vi "HapticSPM_write_test-bench.vi"() -> ()   [LabVIEW 2022 SP3]
uses:
  <vilib>/Utility/sysdir.llb/System Directory Type.ctl
  Haptic-Programming-Interface/LabVIEW VIs/Haptic Prog Interface/Haptic Prog Interface.lvlib
panel:
  out "Signal & Force (Scaled)":dbl[][](graph)
  out "Force vs Signal":cluster{dbl[], dbl[]}(graph)
  in  "Stop":bool
  in  "Mode Selection":string(combo)="2" caption="Combo Box"
  in  "Suggested Settings":bool=TRUE
  in  "Cursor":bool=TRUE
  out "?":bool=TRUE
  out "data":dbl[][](array[numeric])
  in  "Tab Control":enum32{"2 atoms", "1 atom", "Line", "N"}(tab)
  out "Frame Properties (m)":T1
  in  "Function":string(combo)="0" caption="Combo Box"
  in  "Gain (mm/pm)":dbl=2.0 caption="Numeric" format="%.1g"
  in  "k":dbl=0.6000000000000001 caption="Numeric" step=0.1 format="%.1g"
  in  "Setpoint":dbl=8.000000413701856e-11 caption="Numeric" step=1e-11 format="%.0p"
  in  "Gain":dbl=1.0 caption="Numeric" format="%.1g"
  out "Value":dbl caption="Numeric" format="%#_2p"
  out "Click Number":dbl caption="Numeric" format="%#_1g"
  in  "Write Z":bool
  in  "Planing Toggle":bool
  in  "Planing Reset":bool
  in  "Save":bool
  out "Surf Loc (m)":dbl
  out "Forces":T2 {"Fz (N)" format="%.1f"; "Fy (N)" format="%.1f"; "Fx (N)" format="%.1f"}
  out "Position (Reframed)":cluster{"x (m)":dbl, "y (m)":dbl, "z (mm)":dbl} {"z (mm)" format="%.0p"; "y (m)" format="%.1p"; "x (m)" format="%.1p"}
  # "Super Ultra Mega Haptic SPM Controller 3000"
  # "Signal"
  # "Force"
  # "Planing"
  # "Z Write"
  # "Surface Scale"
  # "Move pens in all three dimensions to calibrate\nClick \"enter\" to turn off recommended settings"
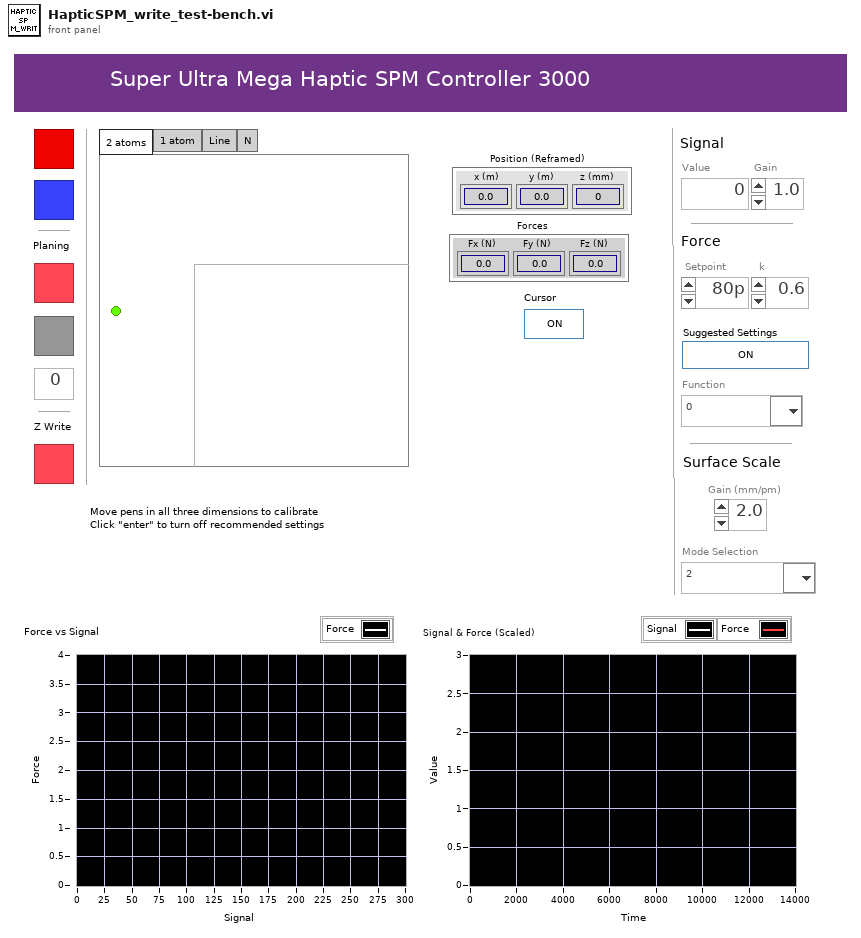
[diagram p1: front panel]
types:
  T1 = cluster{"Origin (m)":cluster{"X Origin (m)":dbl, "Y Origin (m)":dbl}, "Frame Size (m)":cluster{"FW (m)":dbl, "FH (m)":dbl}}
  T2 = cluster{"Fx (N)":dbl, "Fy (N)":dbl, "Fz (N)":dbl}
  T3 = cluster{"kx (N/m)":dbl, "ky (N/m)":dbl, "kz (N/m)":dbl}
  T4 = cluster{"X Drag":bool, "Y Drag":bool, "Z Drag":bool}
  T5 = cluster{"x (mm)":dbl, "y (mm)":dbl, "z (mm)":dbl}
  T6 = typedef "System Directory Type.ctl" = i32
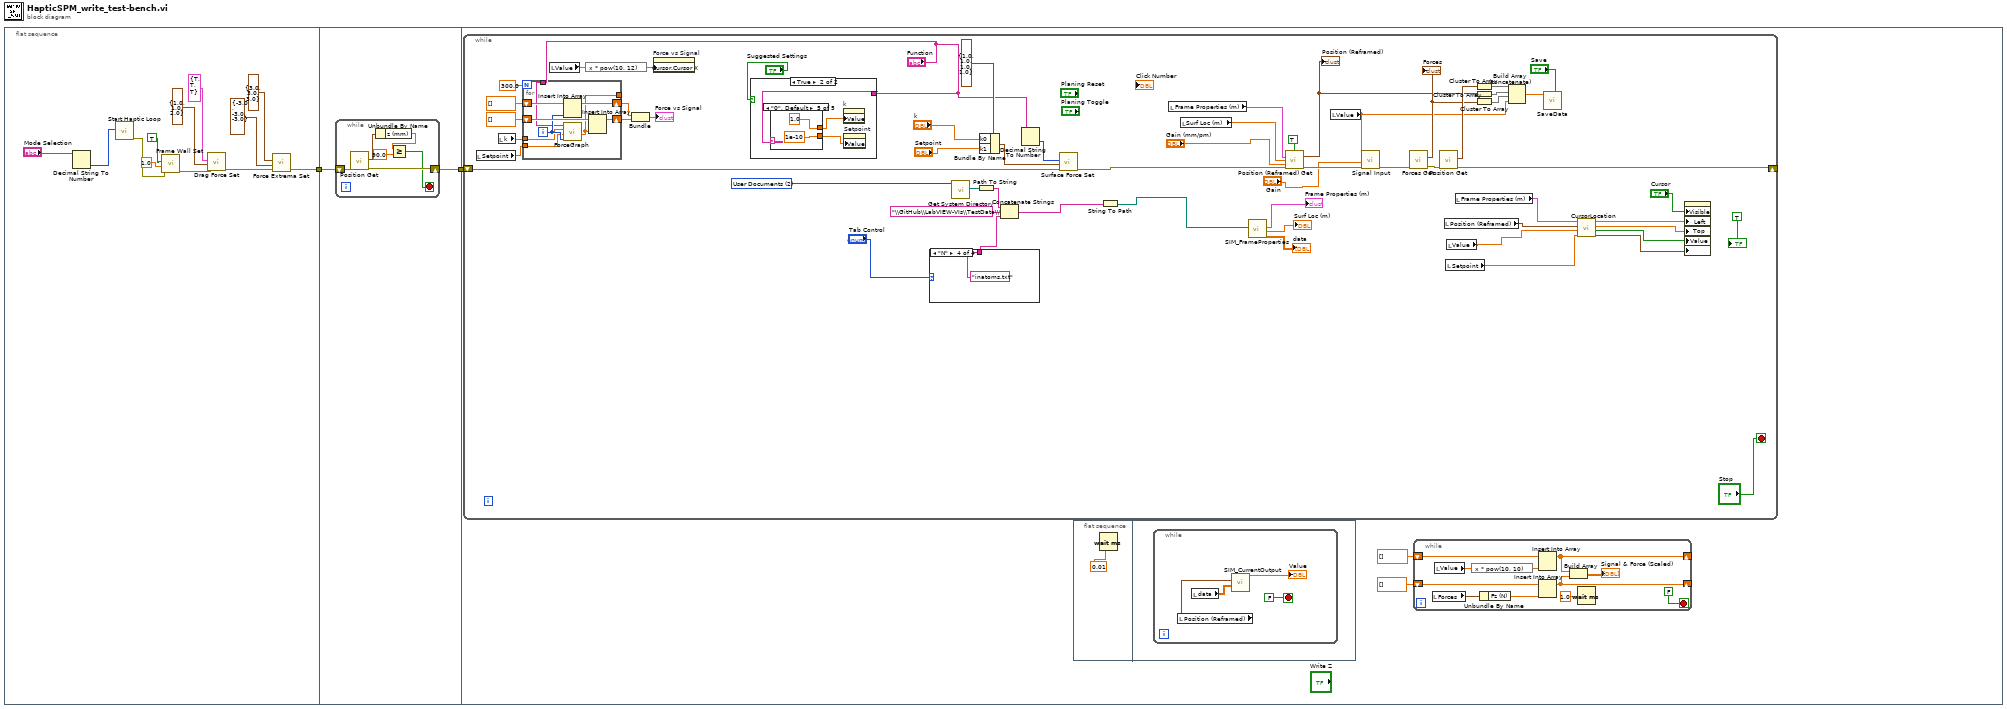
[diagram p0: block diagram]
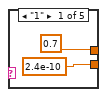
[diagram p3: hidden frame]
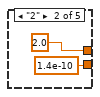
[diagram p4: hidden frame]
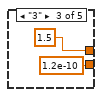
[diagram p5: hidden frame]
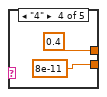
[diagram p6: hidden frame]
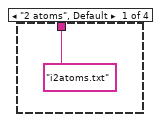
[diagram p7: hidden frame]
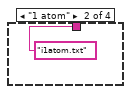
[diagram p8: hidden frame]
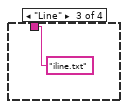
[diagram p9: hidden frame]
diagram:
  n1 = flat-sequence {
    tunnel: [w13] -> w2
    tunnel: w2 -> [w16]
    tunnel: [w15] -> w1
    tunnel: w1 -> [w25]
    frame #0 {
      n2 = Decimal String To Number(string="Mode Selection") -> (number=w3:i32)  [unwired: 2 in, 1 out]
      n3 = call <userlib>:"Start Haptic Loop.vi"("Mode Selection"=w3) -> ("error out"=w5:errorcluster)  [unwired: 10 in]
      n4 = call <userlib>:"Frame Wall Set.vi"("error in (no error)"=w5, "Wall Stiffness (N/m)"=1.0 ("Wall Stiffness"), "Restrict to Frame"=TRUE) -> ("error out"=w6:errorcluster)  [unwired: 8 in]
      n5 = call <userlib>:"Drag Force Set.vi"("error in (no error)"=w6, "Drag Coefficients (N/m)"=T3 {"kx (N/m)"=1.0, "ky (N/m)"=1.0, "kz (N/m)"=2.0} ("Drag Coefficients"), "Drag Force Toggles"=T4 {"X Drag"=TRUE, "Y Drag"=TRUE, "Z Drag"=TRUE}) -> ("error out"=w14:errorcluster)  [unwired: 8 in]
      n6 = call <userlib>:"Force Extrema Set.vi"("error in (no error)"=w14, "Minimum Force (N)"=T2 {"Fx (N)"=-3.0, "Fy (N)"=-3.0, "Fz (N)"=-3.0} ("Minimum Force"), "Maximum Force (N)"=T2 {"Fx (N)"=3.0, "Fy (N)"=3.0, "Fz (N)"=3.0} ("Maximum Force")) -> ("error out"=w13:errorcluster)  [unwired: 8 in]
    }
    frame #1 {
      n7 = while {
        shift-right: [w21] -> w15
        shift-left: w16 -> [w22]
        stop <- w17 stop-if-true
        n8 = call <userlib>:"Position Get.vi"("error in (no error)"=w22) -> ("error out"=w21:errorcluster, "Position"=w20:T5)  [unwired: 9 in]
        n9 = Unbundle By Name(w20) -> ("z (mm)"=w19:dbl)
        n10 = Greater Or Equal?(x=w19, y=90.0) -> (x >= y?=w17:bool)
      }
    }
    frame #2 {
      n11 = while {
        shift-right: [w54] -> _
        shift-left: w25 -> [w100]
        stop <- "Stop" stop-if-true
        w77 = T6 2 items=["User Home"=0, "User Desktop"=1, "User Documents"=2, "User Application Data"=3, "User Preferences"=4, "User Temporary"=5, "Public Documents"=6, "Public Application Data"=7, "Public Preferences"=8, "Public Cache"=13, "System Core Libraries"=9, "System Installed Libraries"=10, "Application Files"=11, "Boot Volume Root"=12] ("system directory type")
        n12 = local read "Setpoint"() -> (w44:dbl)
        n13 = local read "k"() -> (w43:dbl)
        n14 = for {
          N: 300.0 -> [_]
          shift-right: [w109] -> w51
          shift-left: dbl[] [] -> [w107]
          shift-right: [w108] -> w52
          shift-left: dbl[] [] -> [w106]
          tunnel: "Function" -> [w101]
          tunnel: [w104] -> _
          tunnel: w44 -> [w103]
          tunnel: w43 -> [w102]
          i -> [w105]
          n15 = Insert Into Array(array=w106, new element=w105) -> (w108:dbl[])  [unwired: 1 in]
          n16 = call "ForceGraph.vi"("number"=w105, "Setpoint"=w103, "k"=w102, "Function"=w101) -> ("force"=w104:dbl)  [unwired: 7 in]
          n17 = Insert Into Array(array=w107, new element=w104) -> (w109:dbl[])  [unwired: 1 in]
        }
        n18 = local read "Value"() -> (w46:dbl)
        n19 = expression code="x * pow(10, 12)"(w46) -> (w45:dbl)
        n20 = Bundle(w52, w51) -> (→"Force vs Signal":cluster{dbl[], dbl[]})  [unwired: 1 in]
        n21 = property on="Force vs Signal" class="XYGraph (strict)"("Cursor.Cursor X"=w45) -> ()  [unwired: 2 in, 2 out]
        n22 = case shown="True" "Suggested Settings" {
          tunnel: "Function" -> [_ w110]
          frame False {
          }
          frame True {
            n23 = case shown="\"0\", Default" w110 {
              tunnel: [0.7 2.0 1.5 0.4 1.0] -> w112
              tunnel: [2.4e-10 1.4e-10 1.2e-10 8e-11 1e-10] -> w111
              frame "1" {
              }
              frame "2" {
              }
              frame "3" {
              }
              frame "4" {
              }
              frame "0", Default {
              }
            }
            n24 = property on="k" class="DigNum (strict)"("Value"=w112) -> ()  [unwired: 2 in, 2 out]
            n25 = property on="Setpoint" class="DigNum (strict)"("Value"=w111) -> ()  [unwired: 2 in, 2 out]
          }
        }
        n26 = case shown="\"N\"" "Tab Control" {
          tunnel: ["i2atoms.txt" "i1atom.txt" "iline.txt" "inatoms.txt"] -> w58
          frame "2 atoms", Default {
          }
          frame "1 atom" {
          }
          frame "Line" {
          }
          frame "N" {
          }
        }
        n27 = call <vilib>:"Get System Directory.vi"("system directory type"=w77) -> ("system directory"=w76:path)  [unwired: 10 in]
        n28 = Path To String(path=w76) -> (string=w75:string)
        n29 = Bundle By Name(cluster=cluster{"k0":dbl, "k1":dbl, "k2":dbl, "k3":dbl} {"k0"=1.0, "k1"=1.0, "k2"=1.0, "k3"=1.0} ("Force Constants"), "k0"="k", "k1"="Setpoint") -> (w93:cluster{"k0":dbl, "k1":dbl, "k2":dbl, "k3":dbl})
        n30 = Concatenate Strings(w75, "\\GitHub\\LabVIEW-VIs\\TestData\\" ("string"), w58) -> (w73:string)
        n31 = Decimal String To Number(string="Function") -> (number=w92:i32)  [unwired: 2 in, 1 out]
        n32 = call <userlib>:"Surface Force Set.vi"("error in (no error)"=w100, "Force Constants"=w93, "Force Settings"=w92) -> ("error out"=w79:errorcluster)  [unwired: 8 in]
        n33 = String To Path(string=w73) -> (path=w71:path)
        n34 = local read "Frame Properties (m)"() -> (w80:T1)
        n35 = local read "Surf Loc (m)"() -> (w98:dbl)
        n36 = call "SIM_FrameProperties.vi"("file path (dialog if empty)"=w71) -> ("data"=→"data":dbl[][], "Surf Loc (m)"=→"Surf Loc (m)":dbl, "Frame Properties (m)"=→"Frame Properties (m)":T1)  [unwired: 7 in, 1 out]
        n37 = call <userlib>:"Position (Reframed) Get.vi"("Z Rescaling"=TRUE, "Frame Properties (m)"=w80, "Surface Location (m)"=w98, "Scaling (mm per pm)"="Gain (mm/pm)", "error in (no error)"=w79) -> ("Reframed Position (m)"=w70:cluster{"x (m)":dbl, "y (m)":dbl, "z (m)":dbl}, "error out"=w96:errorcluster)  [unwired: 9 in]
        "Position (Reframed)" <- w70
        n38 = local read "Value"() -> (w85:dbl)
        n39 = call <userlib>:"Signal Input.vi"("error in (no error)"=w96, "Gain"="Gain", "Signal"=w85) -> ("error out"=w97:errorcluster)  [unwired: 8 in]
        n40 = call <userlib>:"Forces Get.vi"("error in (no error)"=w97) -> ("error out"=w95:errorcluster, "Force (N)"=w87:T2)  [unwired: 9 in]
        "Forces" <- w87
        n41 = call <userlib>:"Position Get.vi"("error in (no error)"=w95) -> ("error out"=w54:errorcluster, "Position"=w90:T5)  [unwired: 9 in]
        n42 = local read "Position (Reframed)"() -> (w67:cluster{"x (m)":dbl, "y (m)":dbl, "z (mm)":dbl})
        n43 = local read "Setpoint"() -> (w65:dbl)
        n44 = local read "Value"() -> (w66:dbl)
        n45 = local read "Frame Properties (m)"() -> (w68:T1)
        n46 = Cluster To Array(cluster=w90) -> (array=w89:dbl[])
        n47 = Cluster To Array(cluster=w70) -> (array=w88:dbl[])
        n48 = Cluster To Array(cluster=w87) -> (array=w86:dbl[])
        n49 = Build Array (concatenate)(w89, w88, w86, w85) -> (w84:dbl[])
        n50 = call "SaveData.vi"("Save"="Save", "Data"=w84) -> ()  [unwired: 10 in]
        n51 = call "CursorLocation.vi"("Setpoint"=w65, "Value"=w66, "Position (Reframed)"=w67, "Frame Properties (m)"=w68) -> ("Cursor Size"=w61:cluster{"Width":i32, "Height":i32}, "Current Above Setpoint?"=w62:bool, "Y-Coordinate"=w63:dbl, "X-Coordinate"=w64:dbl)
        n52 = property class="Bool (strict)"("Visible"="Cursor", "Left"=w64, "Top"=w63, "Value"=w62, "Button Size"=w61) -> ()  [unwired: 2 in, 2 out]
        "?" <- TRUE
      }
      n53 = flat-sequence {
        frame #0 {
          n54 = Wait (ms)(milliseconds to wait=0.01) -> ()  [unwired: 1 out]
        }
        frame #1 {
          n55 = while {
            stop <- FALSE stop-if-true
            n56 = local read "Position (Reframed)"() -> (w38:cluster{"x (m)":dbl, "y (m)":dbl, "z (mm)":dbl})
            n57 = local read "data"() -> (w39:dbl[][])
            n58 = call "SIM_CurrentOutput.vi"("array"=w39, "Position (Reframed)"=w38) -> ("Current Out (A)"=→"Value":dbl)  [unwired: 8 in, 1 out]
          }
        }
      }
      n59 = while {
        shift-right: [w30] -> _
        shift-left: dbl[] [] ("element") -> [w29]
        shift-right: [w31] -> _
        shift-left: dbl[] [] -> [w32]
        stop <- FALSE stop-if-true
        n60 = local read "Forces"() -> (w28:T2)
        n61 = local read "Value"() -> (w27:dbl)
        n62 = expression code="x * pow(10, 10)"(w27) -> (w34:dbl)
        n63 = Unbundle By Name(w28) -> ("Fz (N)"=w33:dbl)
        n64 = Insert Into Array(array=w29, new element=w34) -> (w30:dbl[])  [unwired: 1 in]
        n65 = Insert Into Array(array=w32, new element=w33) -> (w31:dbl[])  [unwired: 1 in]
        n66 = Build Array(w30, w31) -> (→"Signal & Force (Scaled)":dbl[][])
        n67 = Wait (ms)(milliseconds to wait=1.0) -> ()  [unwired: 1 out]
      }
    }
  }
